vi "IR sensor.vi"(10 "IR sensor shooter raw value":T1, 11 "IR sensor disc":T1) -> ()   [LabVIEW 2012]
uses:
  <vilib>/Rock Robotics/SystemInterfaces/AnalogTrigger/FPGA_AnalogTriggerDevRef.ctl
  <vilib>/Rock Robotics/SystemInterfaces/AnalogTrigger/FPGA_AnalogTriggerIndex.ctl
  Robot Global Data.vi
panel:
  out "Waveform Chart":dbl(graph)
  out "Voltage":dbl
  out "Trigger State":bool
  out "In Window":bool
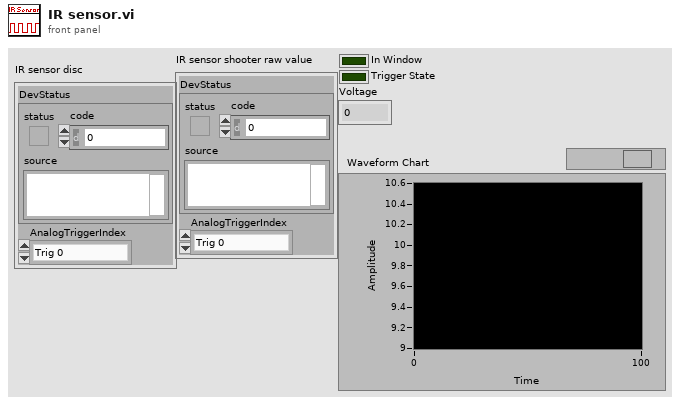
[diagram p1: front panel]
types:
  T1 = typedef "FPGA_AnalogTriggerDevRef.ctl" = cluster{"DevStatus":errorcluster, "AnalogTriggerIndex":T2}
  T2 = typedef "FPGA_AnalogTriggerIndex.ctl" = enum8{"Trig 0", "Trig 1", "Trig 2", "Trig 3", "Trig 4", "Trig 5", "Trig 6", "Trig 7", "Invalid"}
  T3 = typedef "WPI_CounterDevRef.ctl" = cluster{"DevStatus":errorcluster, "CntIndex":T4}
  T4 = typedef "FPGA_CounterCtrSystemIndex.ctl" = enum8{"Ctr 0", "Ctr 1", "Ctr 2", "Ctr 3", "Ctr 4", "Ctr 5", "Ctr 6", "Ctr 7", "Invalid"}
  T5 = typedef "WPI_AnalogChannelDevRef.ctl" = cluster{"DevStatus":errorcluster, "Analog Module":T6, "Analog Channel":T7}
  T6 = typedef "FPGA_TypedefAnalogModule.ctl" = enum16{"Analog Module 1", "Analog Module 2"}
  T7 = typedef "FPGA_AIChannel.ctl" = enum8{"AI 1", "AI 2", "AI 3", "AI 4", "AI 5", "AI 6", "AI 7", "AI 8", "Invalid"}
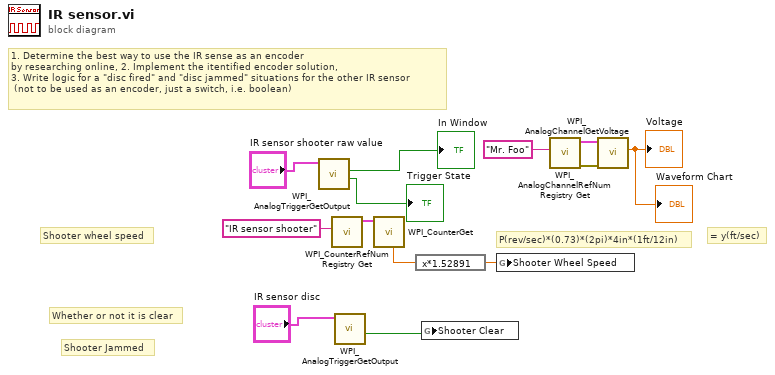
[diagram p0: block diagram]
diagram:
  # "= y(ft/sec)"
  # "Whether or not it is clear"
  # "P(rev/sec)*(0.73)*(2pi)*4in*(1ft/12in)"
  # "Shooter wheel speed"
  # "1. Determine the best way to use the IR sense as an encoder \nby researching online, 2. Implement the itentified encoder solution, \n3. Write logic for a \"disc fired\" and \"disc jammed\" situations for the other IR sensor\n (not to be used as an encoder, just a switch, i.e. boolean)"
  # "Shooter Jammed"
  n1 = call <vilib>:"WPI_AnalogTriggerGetOutput.vi"("AnalogTriggerDevRef"="IR sensor shooter raw value") -> ("Trigger State"=→"Trigger State":bool, "In Window"=→"In Window":bool)  [unwired: 7 in, 2 out]
  n2 = call <vilib>:"WPI_CounterRefNum Registry Get.vi"("refnum name"="IR sensor shooter") -> ("CounterDevRef"=w11:T3)  [unwired: 9 in, 1 out]
  n3 = call <vilib>:"WPI_AnalogTriggerGetOutput.vi"("AnalogTriggerDevRef"="IR sensor disc") -> ("Trigger State"=w8:bool)  [unwired: 7 in, 3 out]
  n4 = call <vilib>:"WPI_CounterGet.vi"("CounterDevRef in"=w11) -> ("Period (sec)"=w13:dbl)  [unwired: 1 in, 9 out]
  n5 = expression code="x*1.52891"(w13) -> (w12:dbl)
  n6 = global write "Robot Global Data.vi" "Shooter Clear"(w8) -> ()
  n7 = global write "Robot Global Data.vi" "Shooter Wheel Speed"(w12) -> ()
  n8 = call <vilib>:"WPI_AnalogChannelRefNum Registry Get.vi"("refnum name"="Mr. Foo") -> ("error out"=w3:errorcluster, "AIDeviceRef"=w2:T5)  [unwired: 9 in]
  n9 = call <vilib>:"WPI_AnalogChannelGetVoltage.vi"("error in (no error)"=w3, "AIDeviceRef"=w2) -> ("Voltage"=→"Waveform Chart" →"Voltage":dbl)  [unwired: 7 in, 2 out]
